vi "Count reset.vi"(8 "error in":errorcluster, 11 "OutputClusterIn":T1={"Acknowledgement"={"Enqueuer"=refnum, "VIReference"=refnum, "VIName"=""}, "AllPartInfo"=[{"PartName"="", "NumberOfRacks"=0, "MeasurementIDsArray"=[], "MeasurementNamesArray"=[], "SpecValuesArray"=[]}], "PartInfo"={"PartName"="", "TotalCount"=0, "ReelCount"=0, "NumberOfRacks"=0, "MeasurementIDsArray"=[], "MeasurementNamesArray"=[], "SpecValuesArray"=[]}, "Result Cluster"={"Measurement Names Array"=[], "Pass-Fail Array"=[], "Measurement Values Array "=[], "Roi for overlay (Arrows) Array"=[], "Algo Type Array"=[], "Image Array"=[], "Clamp operations"=enum."Average Clamp", "  Search Direction "=[], "Images_Array_in"=[], "ResultPF"=FALSE, "Total Cluster Values"={"Total Fail"=0, "Total Pass"=0, "Total Count"=0}, "Reel Counter Cluster"={"Reel Fail"=0, "Reel Pass"=0, "Reel Count"=0}, "Tolerance  Array"=[], "Array of Cam Spec Control Bool"=[], "Control Pass Fail Array"=[], "Specification Pass Fail Array"=[], "Overlay Arrow Lines"=[], "Camera ID"=[], "Trigger count"=0, "Specification fail?"=FALSE}, "ErrorMessage"=""}) -> (0 "error out":errorcluster, 3 "OutputClusterOut":T1={"Acknowledgement"={"Enqueuer"=refnum, "VIReference"=refnum, "VIName"=""}, "AllPartInfo"=[{"PartName"="", "NumberOfRacks"=0, "MeasurementIDsArray"=[], "MeasurementNamesArray"=[], "SpecValuesArray"=[]}], "PartInfo"={"PartName"="", "TotalCount"=0, "ReelCount"=0, "NumberOfRacks"=0, "MeasurementIDsArray"=[], "MeasurementNamesArray"=[], "SpecValuesArray"=[]}, "Result Cluster"={"Measurement Names Array"=[], "Pass-Fail Array"=[], "Measurement Values Array "=[], "Roi for overlay (Arrows) Array"=[], "Algo Type Array"=[], "Image Array"=[], "Clamp operations"=enum."Average Clamp", "  Search Direction "=[], "Images_Array_in"=[], "ResultPF"=FALSE, "Total Cluster Values"={"Total Fail"=0, "Total Pass"=0, "Total Count"=0}, "Reel Counter Cluster"={"Reel Fail"=0, "Reel Pass"=0, "Reel Count"=0}, "Tolerance  Array"=[], "Array of Cam Spec Control Bool"=[], "Control Pass Fail Array"=[], "Specification Pass Fail Array"=[], "Overlay Arrow Lines"=[], "Camera ID"=[], "Trigger count"=0, "Specification fail?"=FALSE}, "ErrorMessage"=""})   [LabVIEW 2019, in "Algorithm.lvclass"]
uses:
  FrameworkOverrides/Algorithm.lvclass
  Controls/Result Cluster.ctl
  Common/Controls/AllPartInfo.ctl
  <vilib>/ActorFramework/Message Enqueuer/Message Enqueuer.lvclass
  Common/Controls/Acknowledgement.ctl
  Controls/OutputCluster.ctl
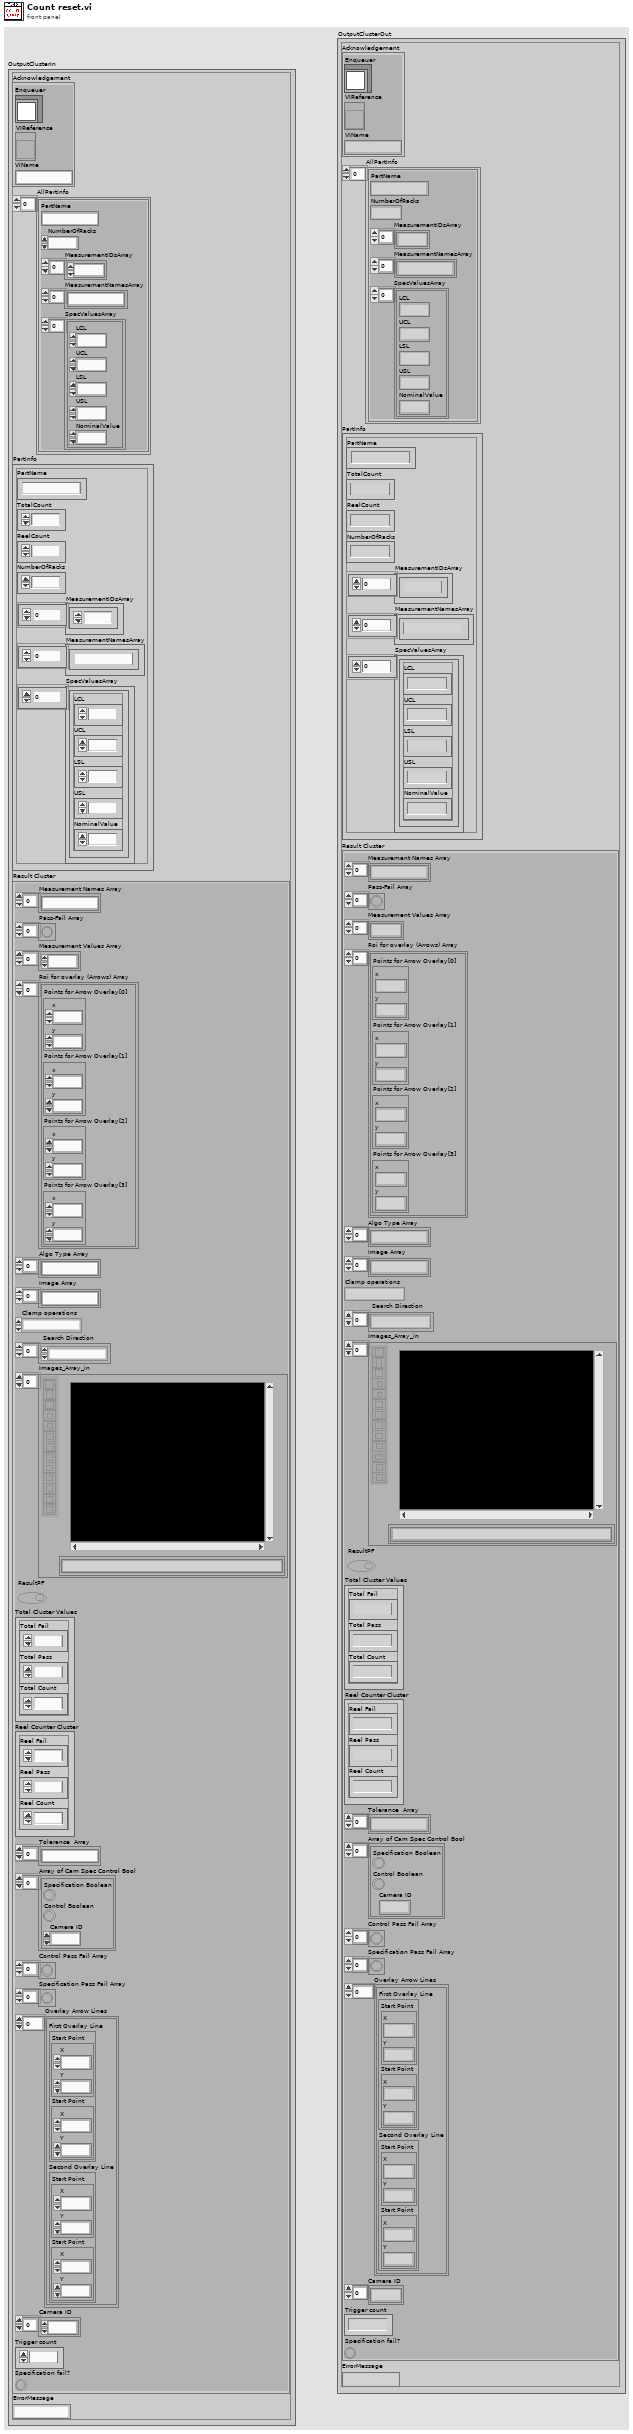
[diagram p1: front panel]
types:
  T1 = typedef "Algorithm.lvclass/OutputCluster.ctl" = cluster{"Acknowledgement":T2, "AllPartInfo":T3, "PartInfo":cluster{"PartName":string, "TotalCount":u64, "ReelCount":u64, "NumberOfRacks":u8, "MeasurementIDsArray":u16[], "MeasurementNamesArray":string[], "SpecValuesArray":cluster{"LCL":dbl, "UCL":dbl, "LSL":dbl, "USL":dbl, "NominalValue":dbl}[]}, "Result Cluster":T4, "ErrorMessage":string}
  T2 = typedef "Acknowledgement.ctl" = cluster{"Enqueuer":refnum<class "Message Enqueuer.lvclass">, "VIReference":refnum<vi>, "VIName":string}
  T3 = typedef "AllPartInfo.ctl" = cluster{"PartName":string, "NumberOfRacks":u8, "MeasurementIDsArray":u16[], "MeasurementNamesArray":string[], "SpecValuesArray":cluster{"LCL":dbl, "UCL":dbl, "LSL":dbl, "USL":dbl, "NominalValue":dbl}[]}[]
  T4 = typedef "Algorithm.lvclass/Result Cluster.ctl" = cluster{"Measurement Names Array":string[], "Pass-Fail Array":bool[], "Measurement Values Array ":dbl[], "Roi for overlay (Arrows) Array":cluster{"Points for Arrow Overlay[0]":cluster{"x":dbl, "y":dbl}, "Points for Arrow Overlay[1]":cluster{"x":dbl, "y":dbl}, "Points for Arrow Overlay[2]":cluster{"x":dbl, "y":dbl}, "Points for Arrow Overlay[3]":cluster{"x":dbl, "y":dbl}}[], "Algo Type Array":string[], "Image Array":string[], "Clamp operations":enum16{"Min Clamp", "Max Clamp", "Average Clamp"}, "  Search Direction ":enum16{"Left to Right", "Right to Left", "Top to Bottom", "Bottom to Top"}[], "Images_Array_in":T5[], "ResultPF":bool, "Total Cluster Values":cluster{"Total Fail":u64, "Total Pass":u64, "Total Count":u64}, "Reel Counter Cluster":cluster{"Reel Fail":u64, "Reel Pass":u64, "Reel Count":u64}, "Tolerance  Array":string[], "Array of Cam Spec Control Bool":cluster{"Specification Boolean":bool, "Control Boolean":bool, "Camera ID":i8}[], "Control Pass Fail Array":bool[], "Specification Pass Fail Array":bool[], "Overlay Arrow Lines":cluster{"First Overlay Line ":cluster{"Start Point":cluster{"X":sgl, "Y":sgl}, "Start Point":cluster{"X":sgl, "Y":sgl}}, "Second Overlay Line ":cluster{"Start Point":cluster{"X":sgl, "Y":sgl}, "Start Point":cluster{"X":sgl, "Y":sgl}}}[], "Camera ID":i8[], "Trigger count":i32, "Specification fail?":bool}
  T5 = typedef "IMAQ Image.ctl" = refnum<image>
  T6 = cluster{"Total Fail":u64, "Total Pass":u64, "Total Count":u64}
  T7 = cluster{"Reel Fail":u64, "Reel Pass":u64, "Reel Count":u64}
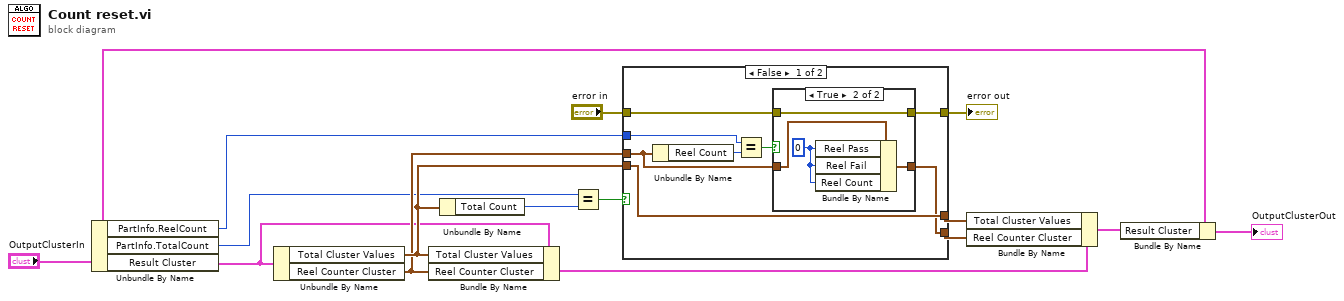
[diagram p0: block diagram]
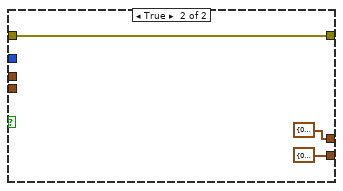
[diagram p3: hidden frame]
diagram:
  n1 = Unbundle By Name("OutputClusterIn") -> ("PartInfo.ReelCount"=w1:u64, "PartInfo.TotalCount"=w2:u64, "Result Cluster"=w6:T4)
  n2 = Unbundle By Name(w6) -> ("Total Cluster Values"=w13:T6, "Reel Counter Cluster"=w10:T7)
  n3 = Bundle By Name(cluster=w6, "Total Cluster Values"=w13, "Reel Counter Cluster"=w10) -> (w9:T4)
  n4 = Unbundle By Name(w13) -> ("Total Count"=w14:u64)
  n5 = Equal?(x=w2, y=w14) -> (x = y?=w15:bool)
  n6 = case shown="False" w15 {
    tunnel: "error in" -> [w19 w32]
    tunnel: [w18 w32] -> w12
    tunnel: w10 -> [w20 _]
    tunnel: [w17 T7 {"Reel Fail"=0, "Reel Pass"=0, "Reel Count"=0} ("Reel Counter Cluster")] -> w7
    tunnel: [w23 T6 {"Total Fail"=0, "Total Pass"=0, "Total Count"=0} ("Total Cluster Values")] -> w8
    tunnel: w13 -> [w23 _]
    tunnel: w1 -> [w16 _]
    frame False {
      n7 = Unbundle By Name(w20) -> ("Reel Count"=w21:u64)
      n8 = Equal?(x=w16, y=w21) -> (x = y?=w22:bool)
      n9 = case shown="True" w22 {
        tunnel: [w24 w29] -> w17
        tunnel: w20 -> [w24 w26]
        tunnel: w19 -> [w25 w28]
        tunnel: [w25 w28] -> w18
        frame False {
        }
        frame True {
          w27 = u64 0 ("Reel Pass-R")
          n10 = Bundle By Name(cluster=w26, "Reel Pass"=w27, "Reel Fail"=w27, "Reel Count"=w27) -> (w29:T7)
        }
      }
    }
    frame True {
    }
  }
  "error out" <- w12
  n11 = Bundle By Name(cluster=w9, "Total Cluster Values"=w8, "Reel Counter Cluster"=w7) -> (w5:T4)
  n12 = Bundle By Name(cluster="OutputClusterIn", "Result Cluster"=w5) -> (→"OutputClusterOut":T1)
